vi "Configure IQ vs Slot Measurement Retrigger.vi"(7 "Retrigger":bool[](array[boolean]), 8 "error in (no error)":errorcluster, 10 "Instance (1)":i32=1, 11 "VISA resource name":refnum<visa-resource-name>) -> (0 "error out":errorcluster, 3 "VISA resource name out":refnum<visa-resource-name>)   [LabVIEW 2020, in "Rohde&Schwarz CMXP GPRF.lvlib"]
doc: "Enables the retrigger mechanism after all frequency/level steps. The setting is relevant for trigger mode \"Retrigger Preselect\".\n\nAttribute:\nRSCMXPGPRF_ATTR_IQ_VS_SLOT_MEASUREMENT_RETRIGGER\n\nRemote-control command:\nCONFigure:GPRF:MEAS<i>:IQVSlot:LIST:RETRigger:ALL"
uses:
  <instrlib>/Rohde&Schwarz CMXP GPRF/Rohde&Schwarz CMXP GPRF.lvlib
  <instrlib>/Rohde&Schwarz CMXP GPRF/Private/rsidr_core.llb/rsidr_core.lvlib
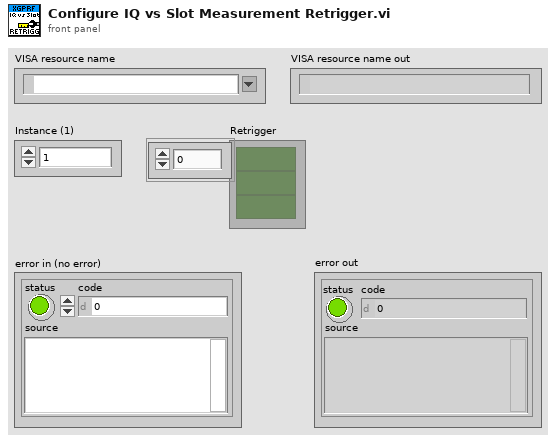
[diagram p1: front panel]
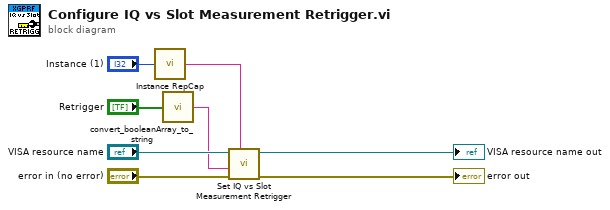
[diagram p0: block diagram]
diagram:
  n1 = call <instrlib>:"Instance RepCap.vi"("Instance in"="Instance (1)") -> ("Instance out"=w2:string)
  n2 = call <instrlib>:"convert_booleanArray_to_string.vi"("Boolean array in"="Retrigger") -> ("string out"=w1:string)  [unwired: 4 in]
  n3 = call "Set IQ vs Slot Measurement Retrigger"("Repeated Capabilities"=w2, "error in (no error)"="error in (no error)", "IQ vs Slot Measurement Retrigger ()"=w1, "instrument handle"="VISA resource name") -> ("error out"=→"error out":errorcluster, "instrument handle out"=→"VISA resource name out":refnum<visa-resource-name>)  [unwired: 6 in]
